vi "GetFrame(SubVI).vi"(1 "pt":T1[](array[typedef])) -> (0 "frame [R T]":dbl[][](array[numeric]) format="%#.2f")   [LabVIEW 2021]
uses:
  ctrOWLMarker.ctl
  <vilib>/Analysis/_algsub.llb/Real Vector Norm.vi
  <vilib>/Analysis/baseanly.llb/Mean (DBL).vi
  <vilib>/Analysis/NI_AALPro.lvlib
  <vilib>/Analysis/NI_AALBase.lvlib
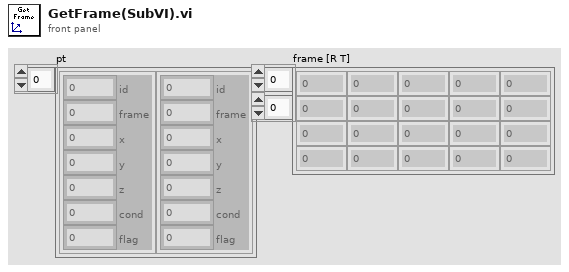
[diagram p1: front panel]
types:
  T1 = typedef "ctrOWLMarker.ctl" = cluster{"id":i32, "frame":i32, "x":sgl, "y":sgl, "z":sgl, "cond":sgl, "flag":u32}
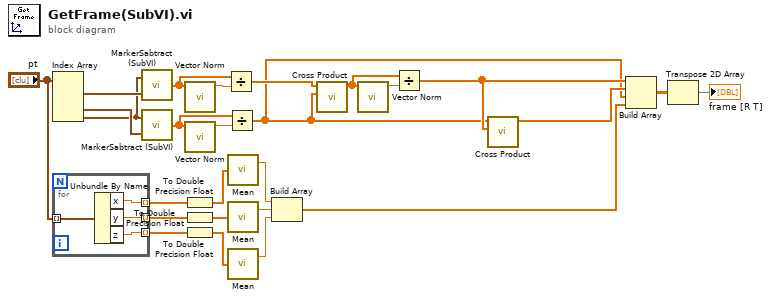
[diagram p0: block diagram]
diagram:
  n1 = Index Array(array="pt") -> (element #1=w7:T1, element #3=w17:T1, element #4=w6:T1)  [unwired: 4 in, 1 out]
  n2 = for {
    tunnel: "pt" -> [w30] mode=indexing
    tunnel: [w29] -> w21 mode=indexing
    tunnel: [w28] -> w22 mode=indexing
    tunnel: [w27] -> w23 mode=indexing
    n3 = Unbundle By Name(w30) -> ("x"=w29:sgl, "y"=w28:sgl, "z"=w27:sgl)
  }
  n4 = call "MarkerSabtract (SubVI).vi"("B"=w7, "A"=w6) -> ("A-B"=w14:dbl[])
  n5 = call "MarkerSabtract (SubVI).vi"("B"=w17, "A"=w6) -> ("A-B"=w11:dbl[])
  n6 = call-poly <vilib>:"Vector Norm.vi"("Input Vector"=w14) -> ("norm"=w13:dbl)  [unwired: 9 in, 1 out]
  n7 = call-poly <vilib>:"Vector Norm.vi"("Input Vector"=w11) -> ("norm"=w12:dbl)  [unwired: 9 in, 1 out]
  n8 = To Double Precision Float(number=w21) -> (double precision float=w18:dbl[])
  n9 = To Double Precision Float(number=w22) -> (double precision float=w19:dbl[])
  n10 = To Double Precision Float(number=w23) -> (double precision float=w20:dbl[])
  n11 = Divide(x=w14, y=w13) -> (x/y=w5:dbl[])
  n12 = Divide(x=w11, y=w12) -> (x/y=w1:dbl[])
  n13 = call-poly <vilib>:"Mean.vi"("X"=w18) -> ("mean"=w24:dbl)  [unwired: 1 out]
  n14 = call-poly <vilib>:"Mean.vi"("X"=w19) -> ("mean"=w25:dbl)  [unwired: 1 out]
  n15 = call-poly <vilib>:"Mean.vi"("X"=w20) -> ("mean"=w26:dbl)  [unwired: 1 out]
  n16 = Build Array(w24, w25, w26) -> (w9:dbl[])
  n17 = call <vilib>:"Cross Product.vi"("B Vector"=w1, "A Vector"=w5) -> ("Cross Product"=w3:dbl[])  [unwired: 8 in, 1 out]
  n18 = call-poly <vilib>:"Vector Norm.vi"("Input Vector"=w3) -> ("norm"=w4:dbl)  [unwired: 9 in, 1 out]
  n19 = Divide(x=w3, y=w4) -> (x/y=w2:dbl[])
  n20 = call <vilib>:"Cross Product.vi"("B Vector"=w2, "A Vector"=w1) -> ("Cross Product"=w15:dbl[])  [unwired: 8 in, 1 out]
  n21 = Build Array(w2, w15, w1, w9) -> (w10:dbl[][])
  n22 = Transpose 2D Array(2D array=w10) -> (transposed array=→"frame [R T]":dbl[][])
